vi "SVT Limit Testing (XY).vi"(8 "error in (no error)":errorcluster, 9 "lower limit":cluster{"X":dbl[], "Y":dbl[]} {"X" format="%.2f"; "Y" format="%.2f"}, 10 "upper limit":cluster{"X":dbl[], "Y":dbl[]} {"X" format="%.2f"; "Y" format="%.2f"}, 11 "signal in":cluster{"X":dbl[], "Y":dbl[]} {"X" format="%.2f"; "Y" format="%.2f"}) -> (0 "error out":errorcluster, 1 "output values":cluster{"frequencies":dbl[], "spectrum":dbl[]}[](graph), 2 "test results":bool[](array[boolean]), 3 "test passed?":bool)   [LabVIEW 2017]
doc: "Performs limit testing on waveforms, spectra, XY data, identified peaks, or scalar measurements. You can wire <B>output values</B> to a graph to view the limits, signal, and failures. You can use this polymorphic VI to perform limit testing of a waveform, a waveform with scalar limits, a spectrum, a spectrum with scalar limits, XY data, XY data with scalar limits, peaks, peaks with scalar limits, or a scalar value. The data type you wire to the <B>signal in</B> input determines the polymorphic instance to use."
uses:
  <vilib>/addons/Sound and Vibration/svt_Limit Test/SoundVib_LimitTest.lvlib
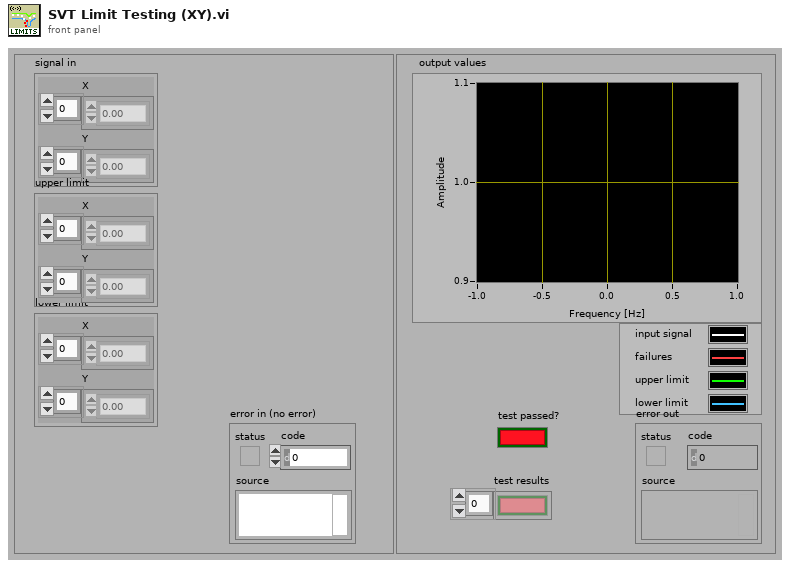
[diagram p1: front panel]
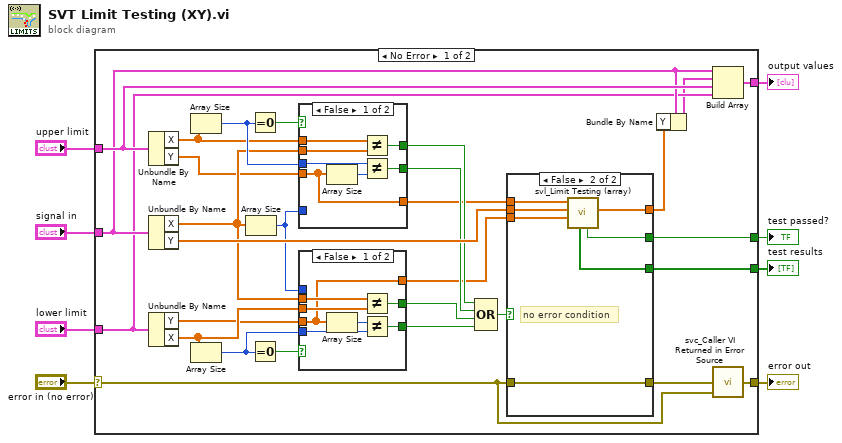
[diagram p0: block diagram]
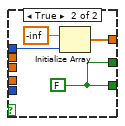
[diagram p2: hidden frame]
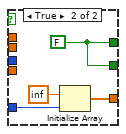
[diagram p3: hidden frame]
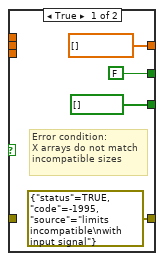
[diagram p4: hidden frame]
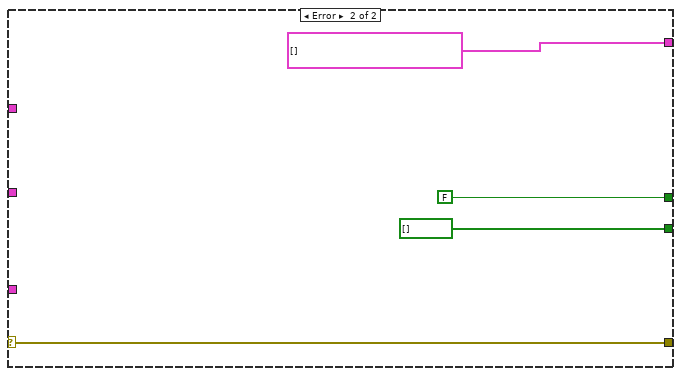
[diagram p5: hidden frame]
diagram:
  n1 = case shown="No Error" "error in (no error)" {
    selector: "error in (no error)" -> [w9 w74]
    tunnel: [w35 w74] -> w7
    tunnel: [w29 bool[] [] ("Array Constant")] -> w6
    tunnel: [w30 FALSE] -> w5
    tunnel: "upper limit" -> [w34 _]
    tunnel: "signal in" -> [w33 _]
    tunnel: "lower limit" -> [w28 _]
    tunnel: [w32 cluster{"X":dbl[], "Y":dbl[]}[] []] -> w1
    frame No Error {
      n2 = Unbundle By Name(w34) -> ("X"=w31:dbl[], "Y"=w14:dbl[])
      n3 = Unbundle By Name(w33) -> ("X"=w15:dbl[], "Y"=w25:dbl[])
      n4 = Unbundle By Name(w28) -> ("Y"=w13:dbl[], "X"=w21:dbl[])
      n5 = Array Size(array=w31) -> (size(s)=w37:i32)
      n6 = Array Size(array=w21) -> (size(s)=w22:i32)
      n7 = Array Size(array=w15) -> (size(s)=w12:i32)
      n8 = Equal To 0?(x=w37) -> (x = 0?=w23:bool)
      n9 = Equal To 0?(x=w22) -> (x = 0?=w20:bool)
      n10 = case shown="False" w23 {
        tunnel: w15 -> [w54 _]
        tunnel: w37 -> [w53 _]
        tunnel: w31 -> [w52 _]
        tunnel: [w51 w59] -> w18
        tunnel: [w50 w59] -> w19
        tunnel: w14 -> [w49 _]
        tunnel: w12 -> [_ w58]
        tunnel: [w49 w56] -> w11
        frame False {
          n11 = Array Size(array=w49) -> (size(s)=w55:i32)
          n12 = Not Equal?(x=w52, y=w54) -> (x != y?=w50:bool)
          n13 = Not Equal?(x=w53, y=w55) -> (x != y?=w51:bool)
        }
        frame True {
          w59 = FALSE
          n14 = Initialize Array(inf ("element"), w58) -> (w56:dbl[])
        }
      }
      n15 = case shown="False" w20 {
        tunnel: w21 -> [w44 _]
        tunnel: w22 -> [w39 _]
        tunnel: w15 -> [w43 _]
        tunnel: [w42 w48] -> w16
        tunnel: [w41 w48] -> w17
        tunnel: w13 -> [w38 _]
        tunnel: w12 -> [_ w47]
        tunnel: [w38 w45] -> w10
        frame False {
          n16 = Array Size(array=w38) -> (size(s)=w40:i32)
          n17 = Not Equal?(x=w43, y=w44) -> (x != y?=w41:bool)
          n18 = Not Equal?(x=w40, y=w39) -> (x != y?=w42:bool)
        }
        frame True {
          w48 = FALSE
          n19 = Initialize Array(-inf ("element"), w47) -> (w45:dbl[])
        }
      }
      n20 = Compound Arithmetic op=OR(w19, w18, w17, w16) -> (w26:bool)
      n21 = case shown="False" w26 {
        tunnel: w9 -> [_ w70]
        tunnel: [errorcluster {"status"=TRUE, "code"=-1995, "source"="limits incompatible\nwith input signal"} ("error IO") w70] -> w36
        tunnel: [dbl[] [] ("failure array") w64] -> w24
        tunnel: [FALSE ("test passed") w66] -> w30
        tunnel: [bool[] [] ("test results") w65] -> w29
        tunnel: w11 -> [_ w69]
        tunnel: w25 -> [_ w68]
        tunnel: w10 -> [_ w67]
        frame True {
          # "Error condition:\nX arrays do not match\nincompatible sizes"
        }
        frame False {
          # "no error condition"
          n22 = call <vilib>:"svl_Limit Testing (array).vi"("lower limit"=w67, "input array"=w68, "upper limit"=w69) -> ("failure array"=w64:dbl[], "test passed"=w66:bool, "test results"=w65:bool[])  [unwired: 4 in, 2 out]
        }
      }
      n23 = Bundle By Name(cluster=w33, "Y"=w24) -> (w27:cluster{"X":dbl[], "Y":dbl[]})
      n24 = Build Array(w33, w27, w34, w28) -> (w32:cluster{"X":dbl[], "Y":dbl[]}[])
      n25 = call <vilib>:"svc_Caller VI Returned in Error Source.vi"("warning input to caller"=w9, "error in (no error)"=w36) -> ("error out"=w35:errorcluster)  [unwired: 3 in]
    }
    frame Error {
    }
  }
  "error out" <- w7
  "output values" <- w1
  "test passed?" <- w5
  "test results" <- w6
